vi "fgv_lidars-databuf.vi"(7 "cmd":enum16{"ini img arr", "write", "read"}(ring), 10 "img-data in":u8[][](array[numeric])) -> (1 "img-data1d out":u8[](array[numeric]), 2 "img-data2d out":u8[][](array[numeric]))   [LabVIEW 2019]
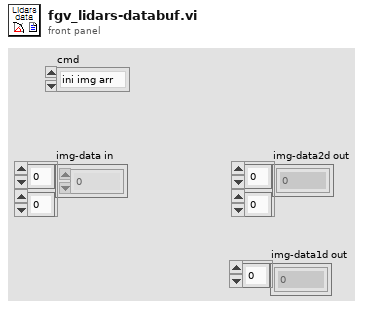
[diagram p1: front panel]
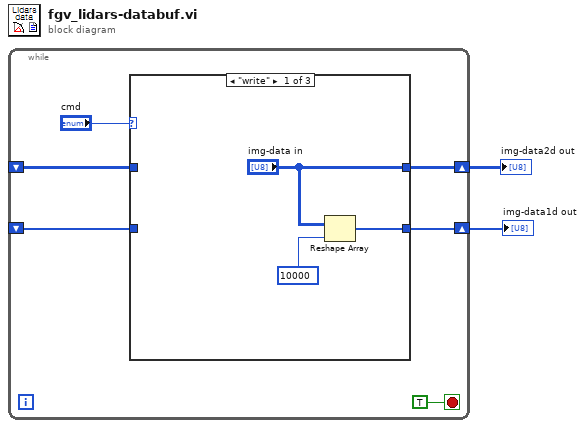
[diagram p0: block diagram]
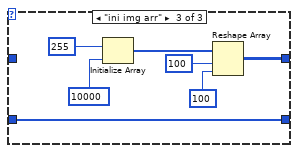
[diagram p3: hidden frame]
diagram:
  n1 = while {
    shift-right: [w6] -> w2
    shift-left: _ -> [w5]
    shift-right: [w4] -> w1
    shift-left: _ -> [w3]
    stop <- TRUE stop-if-true
    n2 = case shown="\"write\"" "cmd" {
      tunnel: ["img-data in" w13 w15] -> w6
      tunnel: w5 -> [_ w13 _]
      tunnel: [w9 w12 w14] -> w4
      tunnel: w3 -> [_ w12 w14]
      frame "write" {
        n3 = Reshape Array("img-data in", 10000 ("dimension size")) -> (w9:u8[])
      }
      frame "read", Default {
      }
      frame "ini img arr" {
        n4 = Initialize Array(u8 255, 10000 ("Constant")) -> (w16:u8[])
        n5 = Reshape Array ("Reshape Array 2")(w16, 100 ("dimension size 3"), 100 ("dimension size 4")) -> (w15:u8[][])
      }
    }
  }
  "img-data2d out" <- w2
  "img-data1d out" <- w1
